vi "unadvertise_close.vi"(8 "连接ID":refnum<k5>, 11 "topic":string) -> ()   [LabVIEW 2014]
panel:
  out "JSON string":string
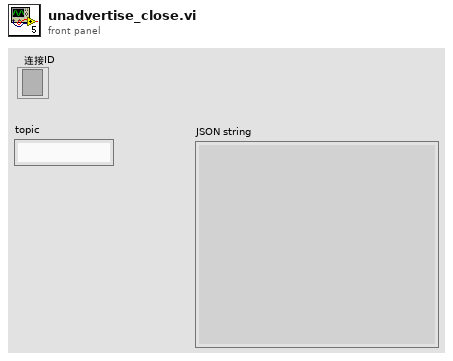
[diagram p1: front panel]
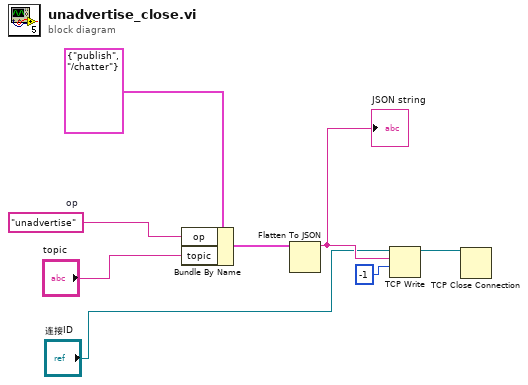
[diagram p0: block diagram]
diagram:
  w6 = "unadvertise"  # op
  n1 = Bundle By Name(cluster=cluster{"op":string, "topic":string} {"op"="publish", "topic"="/chatter"}, "op"=w6, "topic"="topic") -> (w8:cluster{"op":string, "topic":string})
  n2 = Flatten To JSON(anything=w8) -> (JSON string=w4:string)  [unwired: 2 in, 1 out]
  "JSON string" <- w4
  n3 = TCP Write(connection ID="连接ID", data in=w4, 9:-1 ("超时毫秒(25000)")) -> (connection ID out=w1:refnum<k5>)  [unwired: 1 in, 2 out]
  n4 = TCP Close Connection(connection ID=w1) -> ()  [unwired: 2 in, 2 out]
